vi "Apply Scale Options DXF.vi"(6 "Scale Options":T2={"Pos Scale"=1.0, "X Offset"=0.0, "Y Offset"=0.0}, 8 "error in (no error)":errorcluster, 11 "Command Array":T1[](array[typedef])) -> (0 "error out":errorcluster, 3 "Command Array Out":T1[](array[typedef]))   [LabVIEW 2014]
uses:
  Typedefs/DXF Scale Options.ctl
  GCode Parser/GCode Command Cluster.ctl
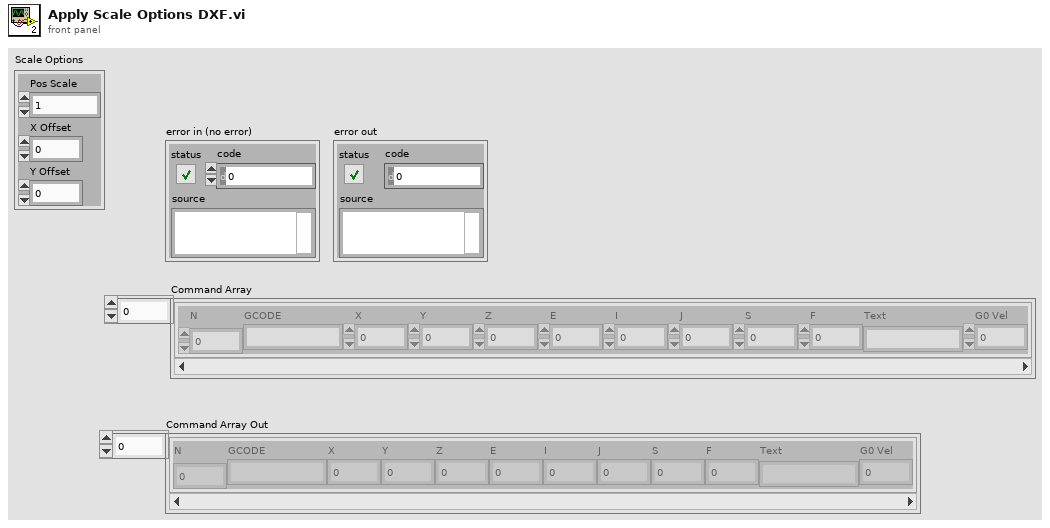
[diagram p1: front panel]
types:
  T1 = typedef "GCode Command Cluster.ctl" = cluster{"N":dbl, "GCODE":string, "X":dbl, "Y":dbl, "Z":dbl, "E":dbl, "I":dbl, "J":dbl, "S":dbl, "F":dbl, "Text":string, "G0 Vel":dbl}
  T2 = typedef "DXF Scale Options.ctl" = cluster{"Pos Scale":dbl, "X Offset":dbl, "Y Offset":dbl}
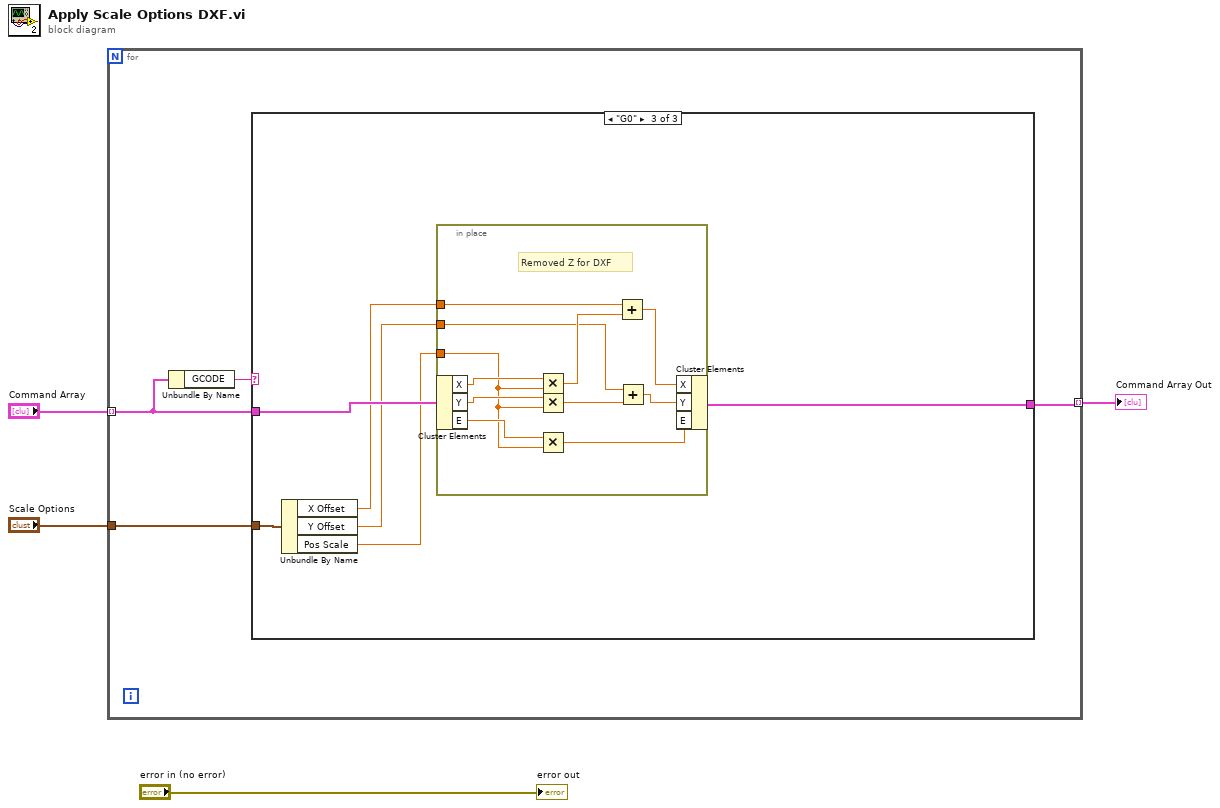
[diagram p0: block diagram]
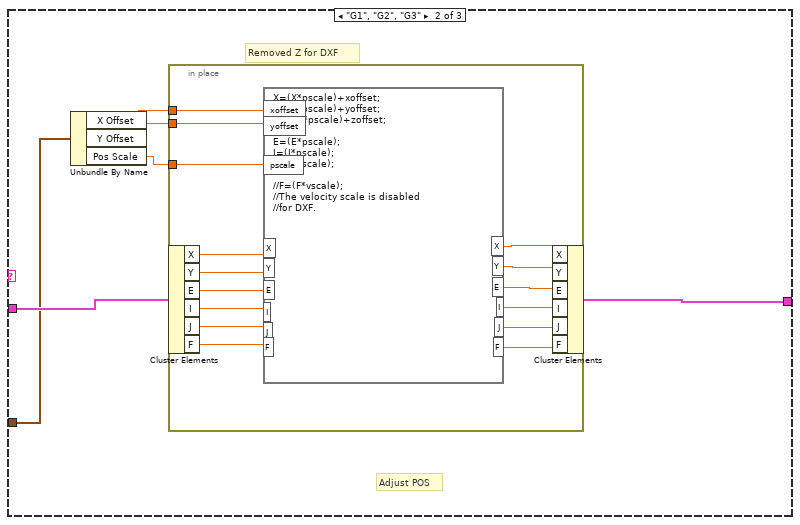
[diagram p3: hidden frame]
diagram:
  n1 = for {
    tunnel: "Scale Options" -> [w7]
    tunnel: "Command Array" -> [w6] mode=indexing
    tunnel: [w5] -> w1 mode=indexing
    n2 = Unbundle By Name(w6) -> ("GCODE"=w8:string)
    n3 = case shown="\"G0\"" w8 {
      tunnel: w6 -> [w9 w15 w36]
      tunnel: [w9 w10 w31] -> w5
      tunnel: w7 -> [_ w14 w35]
      frame "", Default {
      }
      frame "G1", "G2", "G3" {
        # "Removed Z for DXF"
        # "Adjust POS"
        n4 = Unbundle By Name(w14) -> ("X Offset"=w12:dbl, "Y Offset"=w11:dbl, "Pos Scale"=w13:dbl)
        n5 = in-place {
          in-place-border: w13 -> [w18]
          in-place-border: w12 -> [w17]
          in-place-border: w11 -> [w16]
          n6 = in-place-cluster #1(w15) -> ("X"=w30:dbl, "Y"=w29:dbl, "E"=w26:dbl, "I"=w25:dbl, "J"=w28:dbl, "F"=w27:dbl)
          n7 = formula code="X=(X*pscale)+xoffset;\nY=(Y*pscale)+yoffset;\n//Z=(Z*pscale)+zoffset;\n\nE=(E*pscale);\nI=(I*pscale);\nJ=(J*pscale);\n\n//F=(F*vscale);\n//The velocity scale is disabled\n//for DXF."("X"=w30, "Y"=w29, "E"=w26, "I"=w25, "J"=w28, "pscale"=w18, "xoffset"=w17, "yoffset"=w16, "F"=w27) -> ("X"=w24:dbl, "Y"=w23:dbl, "E"=w22:dbl, "I"=w21:dbl, "J"=w20:dbl, "F"=w19:dbl)
          n8 = in-place-cluster #1("X"=w24, "Y"=w23, "E"=w22, "I"=w21, "J"=w20, "F"=w19) -> (w10:T1)
        }
      }
      frame "G0" {
        n9 = Unbundle By Name(w35) -> ("X Offset"=w33:dbl, "Y Offset"=w32:dbl, "Pos Scale"=w34:dbl)
        n10 = in-place {
          in-place-border: w34 -> [w43]
          in-place-border: w33 -> [w40]
          in-place-border: w32 -> [w38]
          # "Removed Z for DXF"
          n11 = in-place-cluster #2(w36) -> ("X"=w47:dbl, "Y"=w46:dbl, "E"=w45:dbl)
          n12 = Multiply(x=w47, y=w43) -> (x*y=w42:dbl)
          n13 = Multiply(x=w46, y=w43) -> (x*y=w37:dbl)
          n14 = Multiply(x=w45, y=w43) -> (x*y=w44:dbl)
          n15 = Add(x=w40, y=w42) -> (x+y=w41:dbl)
          n16 = Add(x=w38, y=w37) -> (x+y=w39:dbl)
          n17 = in-place-cluster #2("X"=w41, "Y"=w39, "E"=w44) -> (w31:T1)
        }
      }
    }
  }
  "Command Array Out" <- w1
  "error out" <- "error in (no error)"
